vi "Evaluate Tag.vi"(8 "error in (no error)":errorcluster, 10 "Tag":string, 11 "XML in":refnum<class "XML.lvclass">) -> (0 "error out":errorcluster, 1 "Tag Name":string, 2 "Header":string, 3 "XML out":refnum<class "XML.lvclass">, 4 "</Tag>":bool, 5 "Attribute":bool)   [LabVIEW 2020, in "XML.lvlib" / "XML.lvclass"]
uses:
  <vilib>/gpm_packages/@cs/persistence/source/XML/XML.lvclass
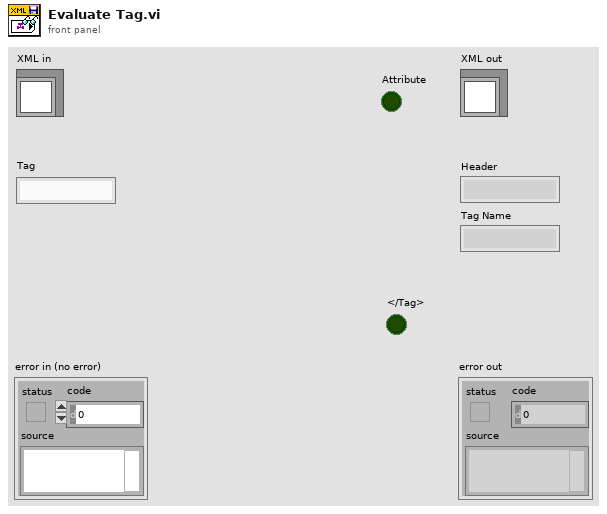
[diagram p1: front panel]
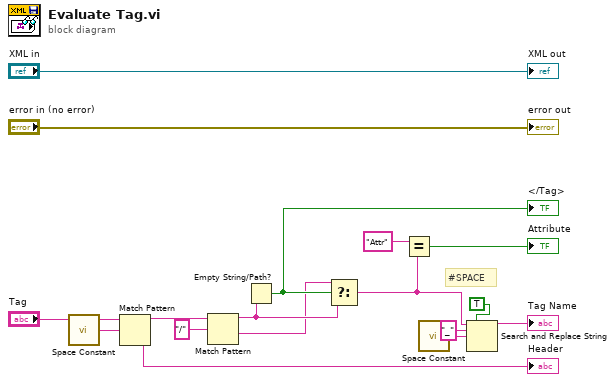
[diagram p0: block diagram]
diagram:
  # "#SPACE"
  n1 = call <vilib>:"Space Constant.vi"() -> ("String"=w17:string)
  n2 = Match Pattern(string="Tag", regular expression=w17) -> (before substring=w14:string, after substring=→"Header":string)  [unwired: 1 in, 2 out]
  n3 = Match Pattern(string=w14, regular expression="/") -> (before substring=w15:string, after substring=w7:string)  [unwired: 1 in, 2 out]
  n4 = Empty String/Path?(string/path=w15) -> (empty?=w12:bool)
  "</Tag>" <- w12
  n5 = Select(t=w7, s=w12, f=w15) -> (s? t:f=w2:string)
  n6 = Equal?(x="Attr", y=w2) -> (x = y?=→"Attribute":bool)
  n7 = call <vilib>:"Space Constant.vi"() -> ("String"=w5:string)
  n8 = Search and Replace String(replace all?=TRUE ("replace all? (F)"), input string=w2, search string="_", replace string=w5) -> (result string=→"Tag Name":string)  [unwired: 4 in, 3 out]
  "error out" <- "error in (no error)"
  "XML out" <- "XML in"
